vi "GetParam.vi"(8 "error in (no error)":errorcluster caption="entrée d'erreur (pas d'erreur)", 11 "Friedman1.lvclass":refnum<class "Friedman1.lvclass">) -> (0 "error out":errorcluster caption="sortie d'erreur", 2 "make_friedman1":T1={"n_samples"=100, "n_features"=10, "noise"=0.0, "random_state"=-1, "Returns"="X"} {"n_features" min=5; "n_samples" min=1}, 3 "Friedman1.lvclass":refnum<class "Friedman1.lvclass">)   [LabVIEW 2020, in "Friedman1.lvclass"]
doc: "Get Parameters"
uses:
  Friedman1.lvclass
  Friedman1.lvclass/Friedman1.ctl
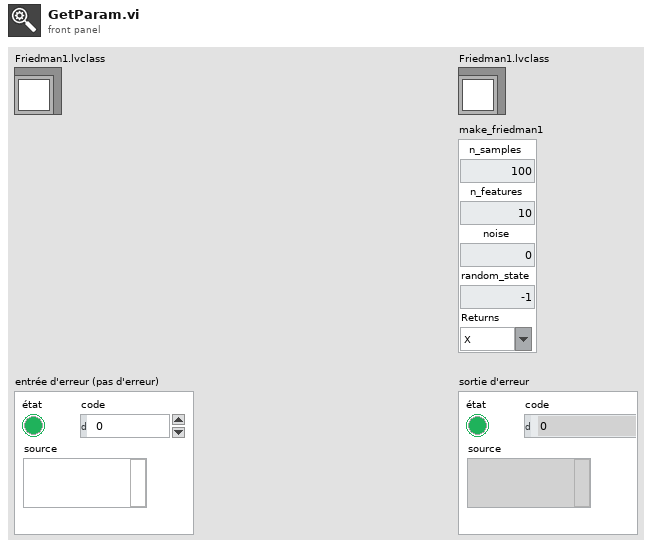
[diagram p1: front panel]
types:
  T1 = cluster{"n_samples":u32, "n_features":u32, "noise":dbl, "random_state":i32, "Returns":string}
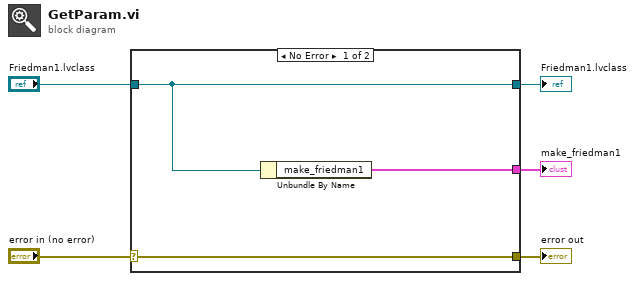
[diagram p0: block diagram]
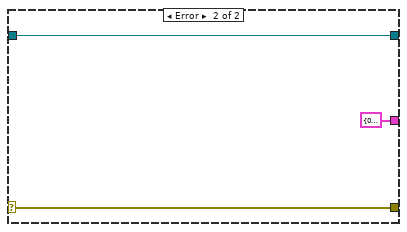
[diagram p2: hidden frame]
diagram:
  n1 = case shown="No Error" "error in (no error)" {
    selector: "error in (no error)" -> [w8 w10]
    tunnel: [w8 w10] -> w4
    tunnel: [w7 w11] -> w2
    tunnel: "Friedman1.lvclass" -> [w7 w11]
    tunnel: [w6 T1 {"n_samples"=0, "n_features"=0, "noise"=0.0, "random_state"=0, "Returns"=""} ("make_friedman1")] -> w1
    frame No Error {
      n2 = Unbundle By Name(w7) -> ("make_friedman1"=w6:T1)
    }
    frame Error {
    }
  }
  "error out" <- w4
  "Friedman1.lvclass" <- w2
  "make_friedman1" <- w1
